vi "GetText.vi"(8 "error in":errorcluster, 11 "node in":refnum<class "sbRIO-9651.lvclass">) -> (0 "error out":errorcluster, 1 "additional text":string, 2 "text":string, 3 "node out":refnum<class "sbRIO-9651.lvclass">, 4 "glyph":string)   [LabVIEW 2014, in "sbRIO-9651.lvclass"]
doc: "Returns the text representation of the node used for the tree control."
uses:
  sbRIO-9651.lvclass
  RIO Target/RIO Target.lvclass
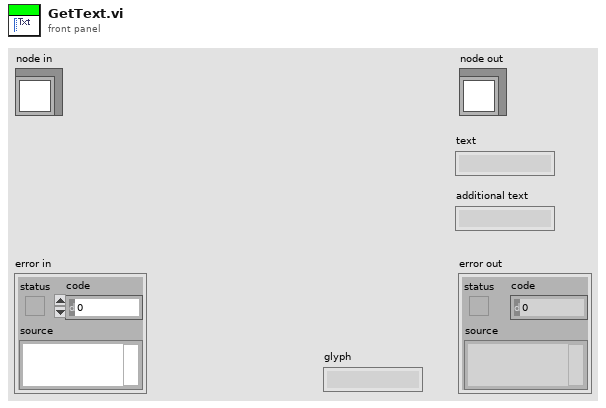
[diagram p1: front panel]
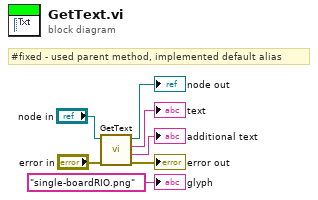
[diagram p0: block diagram]
diagram:
  # "#fixed - used parent method, implemented default alias"
  n1 = call-parent "GetText.vi"("error in"="error in", "node in"="node in") -> ("error out"=→"error out":errorcluster, "additional text"=→"additional text":string, "text"=→"text":string, "node out"=→"node out":refnum<class "sbRIO-9651.lvclass">)  [unwired: 5 in, 1 out]
  "glyph" <- "single-boardRIO.png" ("glyph")
